vi "DFT_normalizado.vi"(11 "X":dbl[](array[numeric])) -> (2 "Array":dbl[](array[numeric]), 3 "Numeric":dbl)   [LabVIEW 2020]
uses:
  <vilib>/Analysis/2dsp.llb/Real FFT.vi
  <vilib>/Analysis/NI_AALPro.lvlib
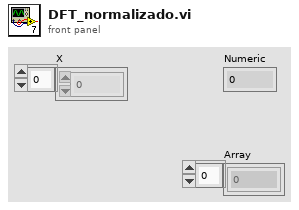
[diagram p1: front panel]
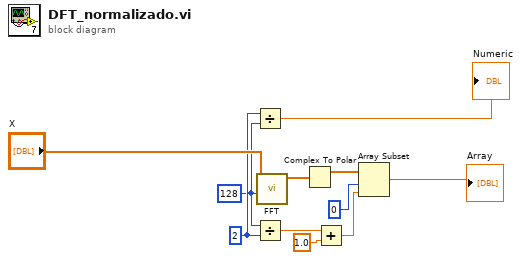
[diagram p0: block diagram]
diagram:
  w2 = 2 ("x")
  w1 = 128 ("FFT size")
  n1 = Divide(x=w2, y=w1) -> (x/y=→"Numeric":dbl)
  n2 = Divide(x=w1, y=w2) -> (x/y=w5:dbl)
  n3 = call-poly <vilib>:"FFT.vi"("FFT size"=w1, "X"="X") -> ("FFT {X}"=w8:cdb[])  [unwired: 8 in, 1 out]
  n4 = Complex To Polar(r * e^(i*theta)=w8) -> (r=w7:dbl[])  [unwired: 1 out]
  n5 = Add(x=w5, y=1.0) -> (x+y=w3:dbl)
  n6 = Array Subset(array=w7, index=0, length=w3) -> (→"Array":dbl[])
